vi "build_parse_tree.vi"(7 "Splitted string tokens":T1, 10 "Splitted string":T3) -> (1 "Root Path":string, 2 "Tree Map Out":T4)   [LabVIEW 2021]
uses:
  <vilib>/National Instruments/Tree Map/Tree Map Data.ctl
  Controls/SplittedString.ctl
  Controls/SplittedStringTokens.ctl
  Controls/Classes.ctl
  <vilib>/National Instruments/Tree Map/Tree Map.lvlib
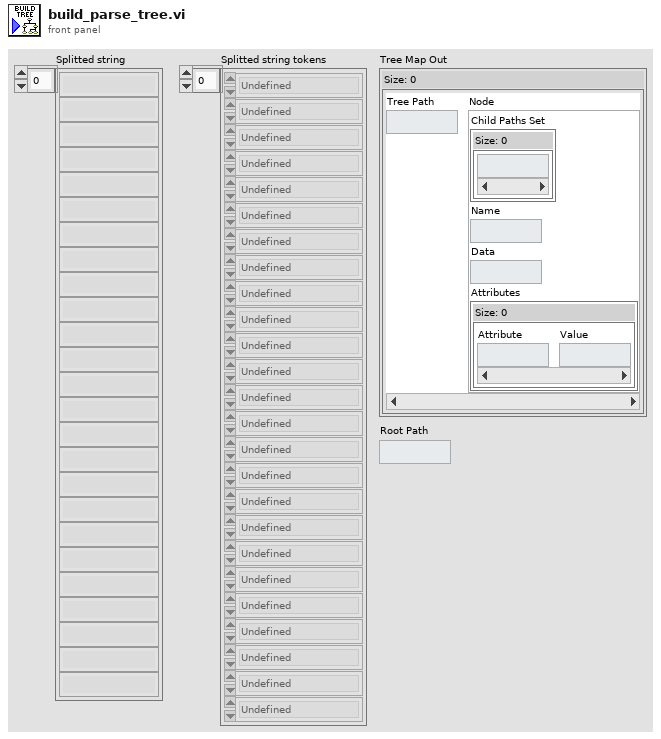
[diagram p1: front panel]
types:
  T1 = typedef "SplittedStringTokens.ctl" = T2[]
  T2 = typedef "Classes.ctl" = enum16{"Undefined", "Left paren", "Right paren", "Number", "Operator", "High level function", "Variable", "End of expression"}
  T3 = typedef "SplittedString.ctl" = string[]
  T4 = typedef "Tree Map.lvlib/Tree Map Data.ctl" = map{string, cluster{"Child Paths Set":set{string}, "Name":string, "Data":string, "Attributes":map{string, string}}}
  T5 = cluster{"Child Paths Set":set{string}, "Name":string, "Data":string, "Attributes":map{string, string}}
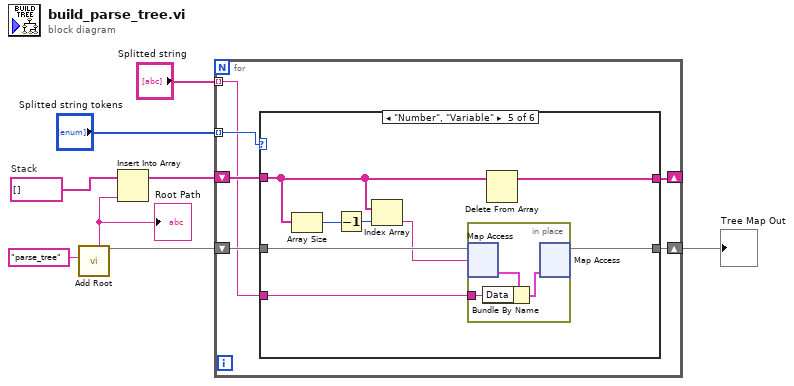
[diagram p0: block diagram]
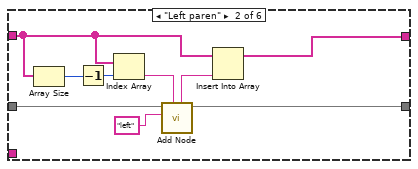
[diagram p3: hidden frame]
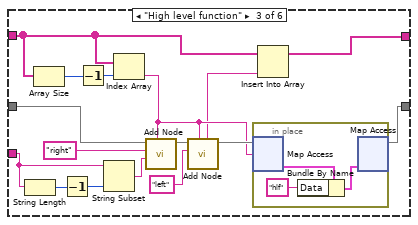
[diagram p4: hidden frame]
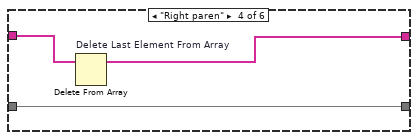
[diagram p5: hidden frame]
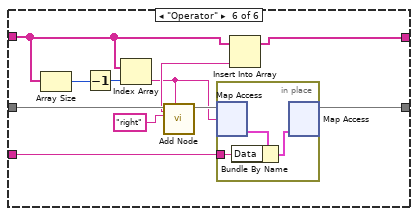
[diagram p6: hidden frame]
diagram:
  w7 = string[] []  # Stack
  n1 = call <vilib>:"Add Root.vi"("New Root Name"="parse_tree") -> ("Tree Map Out"=w5:T4, "Root Path"=w3:string)  [unwired: 9 in]
  "Root Path" <- w3
  n2 = Insert Into Array "Insert Into Array"(array=w7, new element=w3) -> (w6:string[])  [unwired: 1 in]
  n3 = for {
    shift-right: [w11] -> w4
    shift-left: w5 -> [w14]
    shift-right: [w12] -> _
    shift-left: w6 -> [w13]
    tunnel: "Splitted string" -> [w9] mode=indexing
    tunnel: "Splitted string tokens" -> [w10] mode=indexing
    n4 = case shown="\"Number\", \"Variable\"" w10 {
      tunnel: w14 -> [w15 w25 w41 w47 w54 w66]
      tunnel: w13 -> [w16 w20 w38 w46 w49 w63]
      tunnel: [w16 w22 w39 w45 w48 w61] -> w12
      tunnel: [w15 w21 w28 w47 w55 w69] -> w11
      tunnel: w9 -> [_ _ w31 _ w50 w59]
      frame "Undefined", Default {
      }
      frame "Left paren" {
        n5 = Array Size(array=w20) -> (size(s)=w19:i32)
        n6 = Decrement(x=w19) -> (x-1=w18:i32)
        n7 = Index Array "Index Array"(array=w20, index=w18) -> (element=w23:string)
        n8 = call <vilib>:"Add Node.vi"("Parent Path"=w23, "New Node Name"="left", "Tree Map In"=w25) -> ("Tree Map Out"=w21:T4, "New Node Path"=w17:string)  [unwired: 6 in, 1 out]
        n9 = Insert Into Array "Insert Into Array"(array=w20, new element=w17) -> (w22:string[])  [unwired: 1 in]
      }
      frame "High level function" {
        n10 = String Length(string=w31) -> (length=w32:i32)
        n11 = Array Size(array=w38) -> (size(s)=w37:i32)
        n12 = Decrement(x=w32) -> (x-1=w33:i32)
        n13 = Decrement(x=w37) -> (x-1=w36:i32)
        n14 = String Subset(string=w31, length (rest)=w33) -> (substring=w30:string)  [unwired: 1 in]
        n15 = Index Array "Index Array"(array=w38, index=w36) -> (element=w27:string)
        n16 = call <vilib>:"Add Node.vi"("Parent Path"=w27, "Data"=w30, "New Node Name"="right", "Tree Map In"=w41) -> ("Tree Map Out"=w35:T4)  [unwired: 5 in, 2 out]
        n17 = call <vilib>:"Add Node.vi"("Parent Path"=w27, "New Node Name"="left", "Tree Map In"=w35) -> ("Tree Map Out"=w29:T4, "New Node Path"=w26:string)  [unwired: 6 in, 1 out]
        n18 = in-place {
          n19 = in-place-map #1(w29, w27) -> (w43:T5)  [unwired: 1 in, 1 out]
          n20 = Bundle By Name(cluster=w43, "Data"="hlf") -> (w44:T5)
          n21 = in-place-map #1(w44) -> (w28:T4)  [unwired: 1 in, 2 out]
        }
        n22 = Insert Into Array "Insert Into Array"(array=w38, new element=w26) -> (w39:string[])  [unwired: 1 in]
      }
      frame "Right paren" {
        n23 = Delete From Array "Delete Last Element From Array"(array=w46) -> (array with subset deleted=w45:string[])  [unwired: 2 in, 1 out]
      }
      frame "Number", "Variable" {
        n24 = Array Size(array=w49) -> (size(s)=w52:i32)
        n25 = Decrement(x=w52) -> (x-1=w53:i32)
        n26 = Index Array "Index Array"(array=w49, index=w53) -> (element=w51:string)
        n27 = in-place {
          in-place-border: w50 -> [w56]
          n28 = in-place-map #2(w54, w51) -> (w57:T5)  [unwired: 1 in, 1 out]
          n29 = Bundle By Name(cluster=w57, "Data"=w56) -> (w58:T5)
          n30 = in-place-map #2(w58) -> (w55:T4)  [unwired: 1 in, 2 out]
        }
        n31 = Delete From Array "Delete From Array"(array=w49) -> (array with subset deleted=w48:string[])  [unwired: 2 in, 1 out]
      }
      frame "Operator" {
        n32 = Array Size(array=w63) -> (size(s)=w67:i32)
        n33 = Decrement(x=w67) -> (x-1=w68:i32)
        n34 = Index Array "Index Array"(array=w63, index=w68) -> (element=w60:string)
        n35 = call <vilib>:"Add Node.vi"("Parent Path"=w60, "New Node Name"="right", "Tree Map In"=w66) -> ("Tree Map Out"=w65:T4, "New Node Path"=w62:string)  [unwired: 6 in, 1 out]
        n36 = in-place {
          in-place-border: w59 -> [w70]
          n37 = in-place-map #3(w65, w60) -> (w71:T5)  [unwired: 1 in, 1 out]
          n38 = Bundle By Name(cluster=w71, "Data"=w70) -> (w72:T5)
          n39 = in-place-map #3(w72) -> (w69:T4)  [unwired: 1 in, 2 out]
        }
        n40 = Insert Into Array "Insert Into Array"(array=w63, new element=w62) -> (w61:string[])  [unwired: 1 in]
      }
    }
  }
  "Tree Map Out" <- w4
